vi "操作Sql的Sample-simple.vi"(3 "SavefileName":string="\\\\192.168.20.200\\立讯精密\\工程部\\电子&测试工程课\\临时文件\\WMG\\1. 源程序\\3. EEPROM Test_Rev2.0\\EEPROM Code\\L0000-110\\L0000-110.txt", 5 "DB":T1, 6 "sn 2":string="L0000-110", 7 "fieldName":string="MapFile", 8 "下载文件":bool=TRUE, 9 "fileName":string="C:\\9999.txt", 10 "fieldName_Index":string="S4P10G", 11 "sn":string="SFP+ 002") -> ()   [LabVIEW 2011]
uses:
  Data/ClassLibrary_Sql 1.2.dll
panel:
  out "UpdateStreamFileToSql":bool
  out "StreamFileToSql":bool
  in  "fieldName_Sn 2":string="PN"
  in  "fieldName_Sn":string="FixtureNo"
  in  "tableName":string="EEPROMManagement"
  out "GetFileFromSql":bool
  out "SelectTheRecordIsExist 2":bool
  out "SelectTheRecordIsExist":bool
  # "查询和上传文件"
  # "固定，表名"
  # "固定，列名"
  # "固定，列名"
  # "查询和下载文件"
  # "固定，列名"
  # "固定，列名"
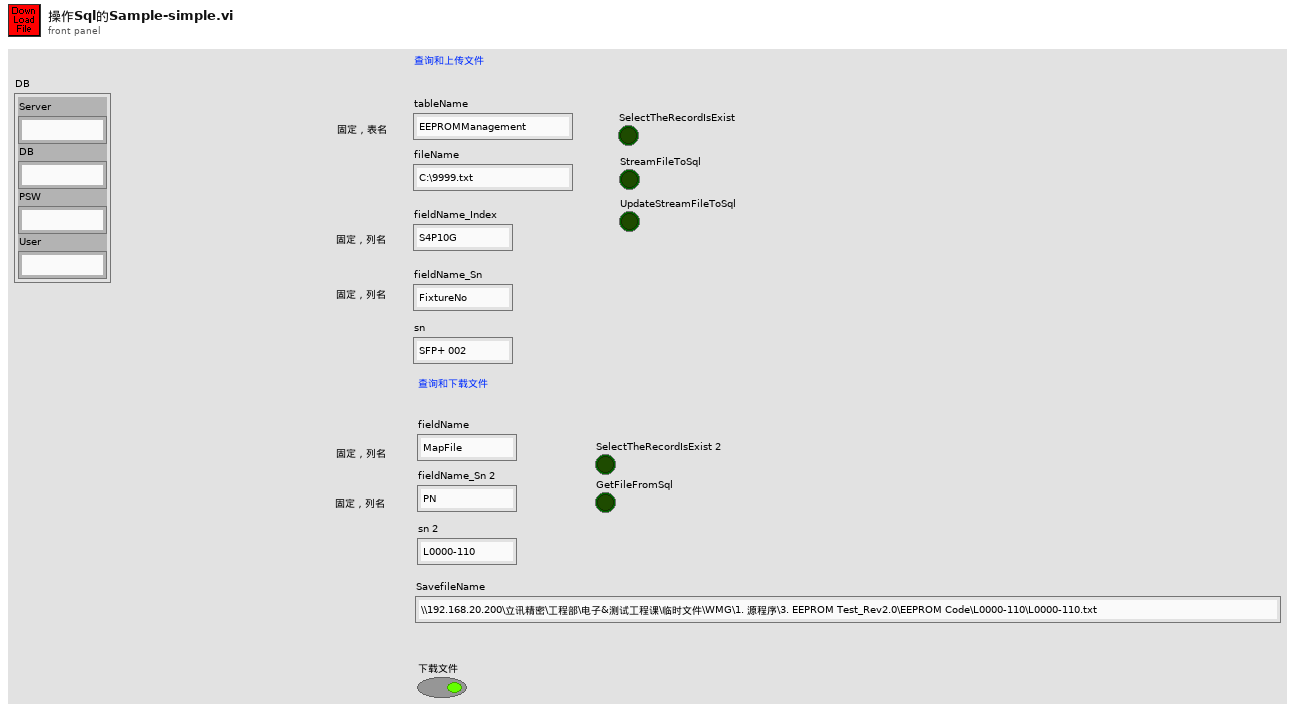
[diagram p1: front panel]
types:
  T1 = cluster{"Server":string, "DB":string, "PSW":string, "User":string}
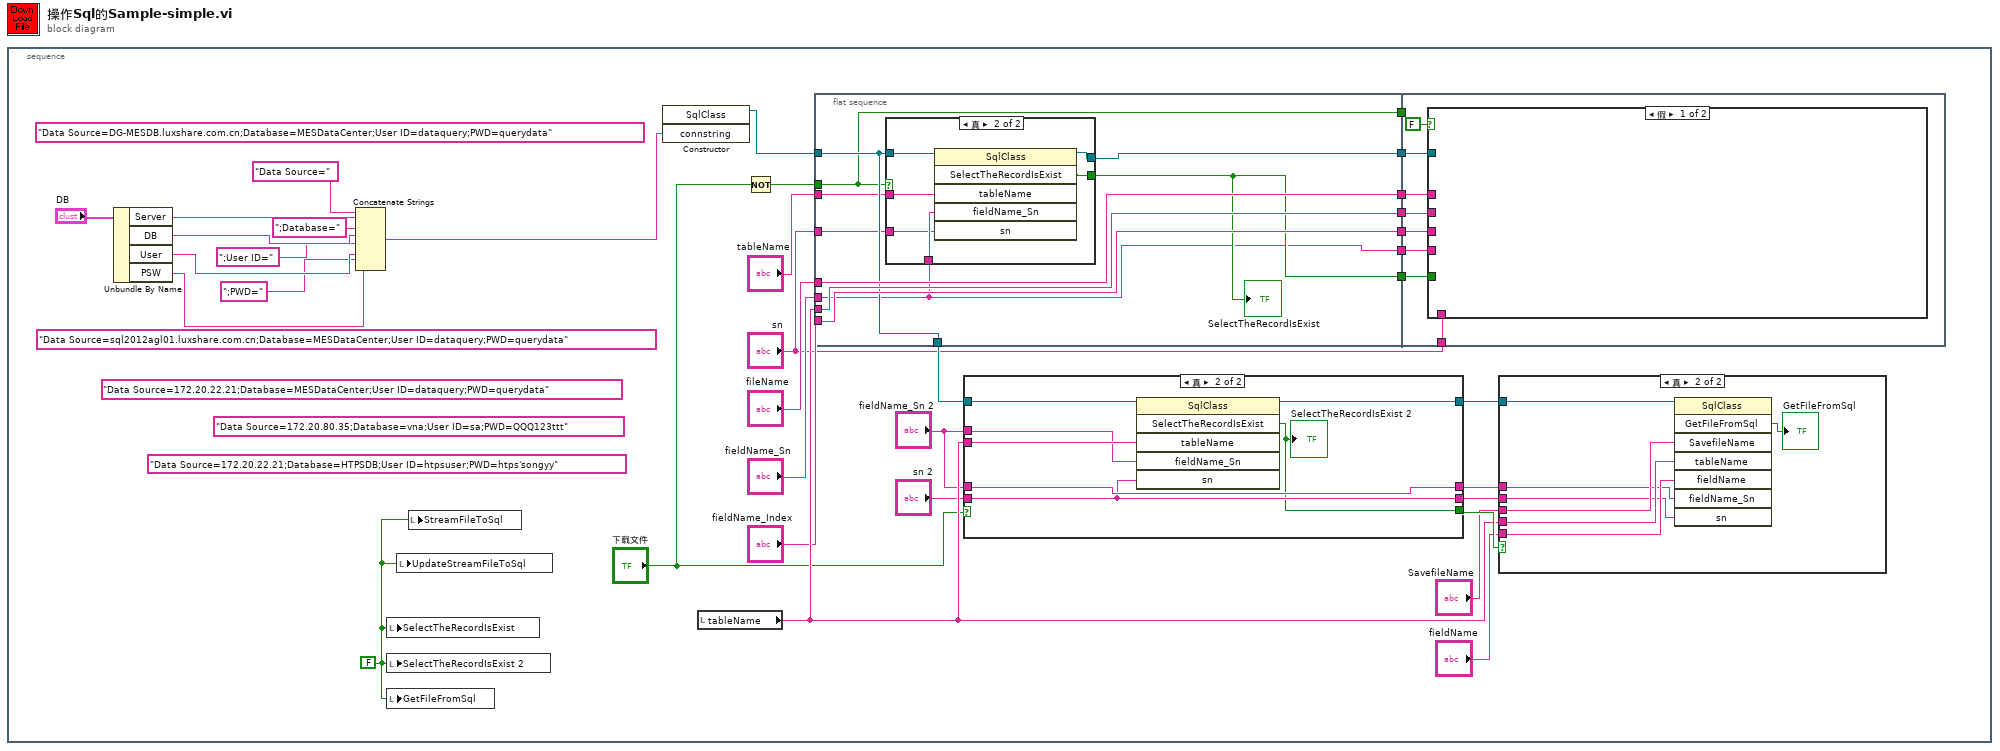
[diagram p0: block diagram]
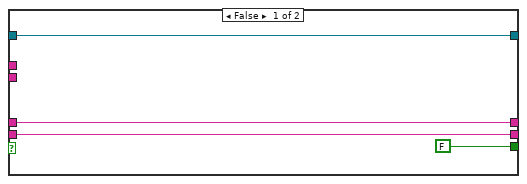
[diagram p3: hidden frame]
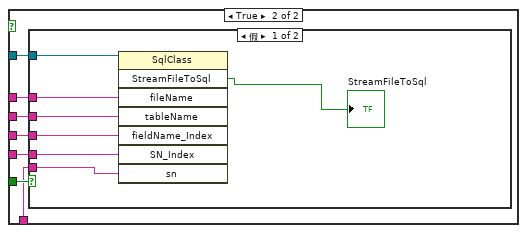
[diagram p5: hidden frame]
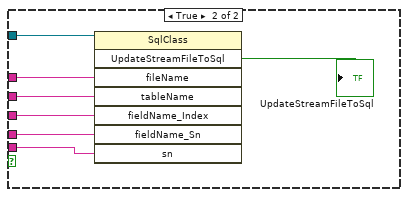
[diagram p6: hidden frame]
diagram:
  n1 = stacked-sequence {
    frame #0 {
      (unwired) "Data Source=sql2012agl01.luxshare.com.cn;Database=MESDataCenter;User ID=dataquery;PWD=querydata" ("connstring")
      (unwired) "Data Source=172.20.22.21;Database=MESDataCenter;User ID=dataquery;PWD=querydata" ("connstring")
      (unwired) "Data Source=172.20.22.21;Database=HTPSDB;User ID=htpsuser;PWD=htps'songyy" ("connstring")
      (unwired) "Data Source=172.20.80.35;Database=vna;User ID=sa;PWD=QQQ123ttt" ("connstring")
      w14 = FALSE
      (unwired) "Data Source=DG-MESDB.luxshare.com.cn;Database=MESDataCenter;User ID=dataquery;PWD=querydata" ("connstring")
      n2 = Unbundle By Name("DB") -> ("Server"=w8:string, "DB"=w6:string, "User"=w4:string, "PSW"=w2:string)
      n3 = Concatenate Strings("Data Source=" ("字符串"), w8, ";Database=" ("字符串"), w6, ";User ID=" ("字符串"), w4, ";PWD=" ("字符串"), w2) -> (w1:string)
      n4 = local write "SelectTheRecordIsExist"(w14) -> ()
      n5 = local write "SelectTheRecordIsExist 2"(w14) -> ()
      n6 = local write "GetFileFromSql"(w14) -> ()
      n7 = local write "UpdateStreamFileToSql"(w14) -> ()
      n8 = local write "StreamFileToSql"(w14) -> ()
      n9 = constructor class="SqlClass"("connstring"=w1) -> (reference out=w13:refnum<k24>)  [unwired: 3 in, 3 out]
      n10 = local read "tableName"() -> (w25:string)
      n11 = Not(x="下载文件") -> (.not. x?=w12:bool)
      n12 = flat-sequence {
        tunnel: [w59] -> w36
        tunnel: [w61] -> w29
        tunnel: "tableName" -> [w58]
        tunnel: w25 -> [w63]
        tunnel: [w63] -> w35
        tunnel: "fileName" -> [w62]
        tunnel: [w62] -> w34
        tunnel: "fieldName_Index" -> [w64]
        tunnel: [w64] -> w33
        tunnel: "fieldName_Sn" -> [w57]
        tunnel: [w57] -> w32
        tunnel: "sn" -> [w56]
        tunnel: [w60] -> w31
        tunnel: w13 -> [w61]
        tunnel: w12 -> [w55]
        tunnel: [w55] -> w30
        tunnel: w36 -> [w78]
        tunnel: w35 -> [w77]
        tunnel: w34 -> [w76]
        tunnel: w33 -> [w75]
        tunnel: w32 -> [w74]
        tunnel: "sn" -> [w73]
        tunnel: w31 -> [w72]
        tunnel: w30 -> [_]
        frame #0 {
          n13 = case shown="真" w55 {
            tunnel: w61 -> [_ w70]
            tunnel: [_ w69] -> w60
            tunnel: [_ w68] -> w59
            tunnel: w58 -> [_ w67]
            tunnel: w57 -> [_ w66]
            tunnel: w56 -> [_ w65]
            frame False {
            }
            frame True {
              n14 = invoke class="SqlClass" method="SelectTheRecordIsExist"(reference=w70, "tableName"=w67, "fieldName_Sn"=w66, "sn"=w65) -> (reference out=w69:refnum<k24>, "SelectTheRecordIsExist"=w68:bool)  [unwired: 2 in, 4 out]
            }
          }
          "SelectTheRecordIsExist" <- w59
        }
        frame #1 {
          n15 = case shown="假" FALSE {
            tunnel: w78 -> [_ w85]
            tunnel: w77 -> [_ w84]
            tunnel: w76 -> [_ w83]
            tunnel: w75 -> [_ w82]
            tunnel: w74 -> [_ w81]
            tunnel: w73 -> [_ w80]
            tunnel: w72 -> [_ w79]
            frame False {
            }
            frame True {
              n16 = case shown="假" w85 {
                tunnel: w84 -> [w90 w97]
                tunnel: w83 -> [w91 w98]
                tunnel: w82 -> [w88 w96]
                tunnel: w81 -> [w87 w95]
                tunnel: w80 -> [w89 w94]
                tunnel: w79 -> [w92 w99]
                frame False {
                  n17 = invoke class="SqlClass" method="StreamFileToSql"(reference=w92, "fileName"=w91, "tableName"=w90, "fieldName_Index"=w88, "SN_Index"=w87, "sn"=w89) -> ("StreamFileToSql"=→"StreamFileToSql":bool)  [unwired: 2 in, 7 out]
                }
                frame True {
                  n18 = invoke class="SqlClass" method="UpdateStreamFileToSql"(reference=w99, "fileName"=w98, "tableName"=w97, "fieldName_Index"=w96, "fieldName_Sn"=w95, "sn"=w94) -> ("UpdateStreamFileToSql"=→"UpdateStreamFileToSql":bool)  [unwired: 2 in, 7 out]
                }
              }
            }
          }
        }
      }
      n19 = case shown="真" "下载文件" {
        tunnel: w29 -> [w46 w53]
        tunnel: [FALSE ("SelectTheRecordIsExist") w49] -> w28
        tunnel: [w46 w48] -> w27
        tunnel: w25 -> [_ w52]
        tunnel: "fieldName_Sn 2" -> [_ w51]
        tunnel: "sn 2" -> [w45 w50]
        tunnel: [w47 w54] -> w20
        tunnel: "fieldName_Sn 2" -> [w47 w54]
        tunnel: [w45 w50] -> w18
        frame False {
        }
        frame True {
          n20 = invoke class="SqlClass" method="SelectTheRecordIsExist"(reference=w53, "tableName"=w52, "fieldName_Sn"=w51, "sn"=w50) -> (reference out=w48:refnum<k24>, "SelectTheRecordIsExist"=w49:bool)  [unwired: 2 in, 4 out]
          "SelectTheRecordIsExist 2" <- w49
        }
      }
      n21 = case shown="真" w28 {
        tunnel: w27 -> [_ w43]
        tunnel: w25 -> [_ w41]
        tunnel: w20 -> [_ w39]
        tunnel: "fieldName" -> [_ w40]
        tunnel: w18 -> [_ w38]
        tunnel: "SavefileName" -> [_ w42]
        frame False {
        }
        frame True {
          n22 = invoke class="SqlClass" method="GetFileFromSql"(reference=w43, "SavefileName"=w42, "tableName"=w41, "fieldName"=w40, "fieldName_Sn"=w39, "sn"=w38) -> ("GetFileFromSql"=→"GetFileFromSql":bool)  [unwired: 2 in, 7 out]
        }
      }
    }
  }
